vi "setAttribute.vi"(8 "error in (no error)":errorcluster, 10 "Emissivity":dbl, 11 "ax5.lvclass":refnum<class "ax5.lvclass">) -> (0 "error out":errorcluster, 3 "ax5.lvclass":refnum<class "ax5.lvclass">)   [LabVIEW 2017, in "ax5.lvclass"]
uses:
  ax5.lvclass
  \\psf\Home/Desktop/Elkhorn Test/Elkhorn Test/JSONRPC Server Framework Examples/builds/JSON RPC over TCP/RT CompactRIO Target/My Source Distribution/home/lvuser/natinst/bin/methods/camera.lvclass
  <resource>/objmgr/imaqdx.rc
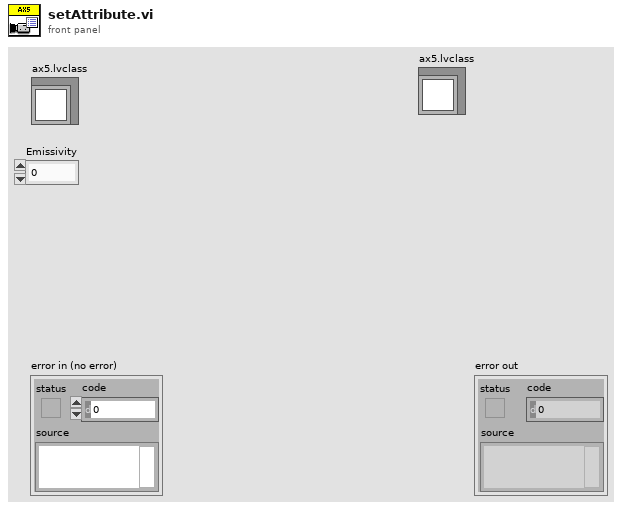
[diagram p1: front panel]
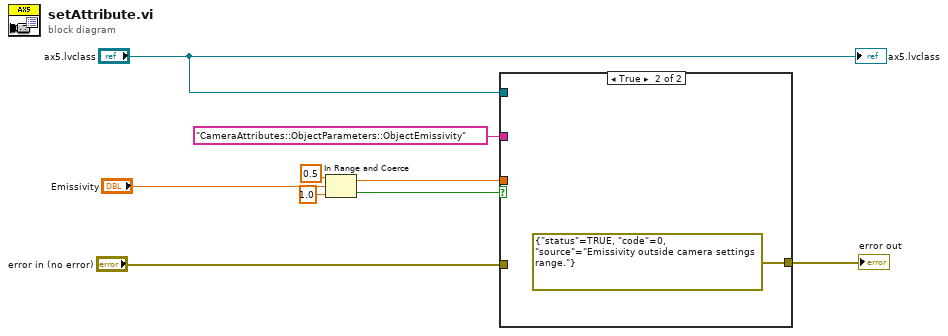
[diagram p0: block diagram]
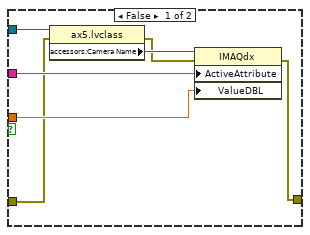
[diagram p2: hidden frame]
diagram:
  n1 = In Range and Coerce(upper limit=0.5, x="Emissivity", lower limit=1.0) -> (coerced(x)=w5:dbl, In Range?=w3:bool)
  n2 = case shown="True" w3 {
    tunnel: "ax5.lvclass" -> [w16 _]
    tunnel: w5 -> [w13 _]
    tunnel: "CameraAttributes::ObjectParameters::ObjectEmissivity" -> [w12 _]
    tunnel: "error in (no error)" -> [w11 _]
    tunnel: [w10 errorcluster {"status"=TRUE, "code"=0, "source"="Emissivity outside camera settings range."} ("error out")] -> w1
    frame False {
      n3 = property class="ax5.lvclass"(reference=w16, error in=w11) -> (error out=w14:errorcluster, "accessors:Camera Name"=w15:refnum<k21>)  [unwired: 1 out]
      n4 = property class="IMAQdx"(reference=w15, error in=w14, "ActiveAttribute"=w12, "ValueDBL"=w13) -> (error out=w10:errorcluster)  [unwired: 1 out]
    }
    frame True {
    }
  }
  "error out" <- w1
  "ax5.lvclass" <- "ax5.lvclass"
